vi "Write Size.vi"(10 "Size":dbl, 11 "Movable in":refnum<class "Movable.lvclass">) -> (3 "Movable out":refnum<class "Movable.lvclass">)   [LabVIEW 2021, in "Movable.lvclass"]
doc: "MIT Licence\nCopyright (c) 2024 David Grollier"
uses:
  Movable.lvclass
  Movable.lvclass/Movable.ctl
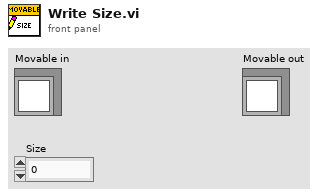
[diagram p1: front panel]
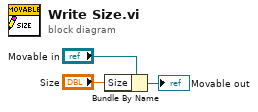
[diagram p0: block diagram]
diagram:
  n1 = Bundle By Name(cluster="Movable in", "Size"="Size") -> (→"Movable out":refnum<class "Movable.lvclass">)
